vi "AMI Get 2D field (Polar).vi"(8 "error in":T2, 10 "Z-Axis Communications Config":T1={"GPIB address"=22, "GPIB bus"=0, "connection ID"=refnum, "IP"="192.168.2.200", "Active Comm Interface"=0, "Serial Port"="", "Programmer Type"=0} {"Programmer Type" items=["Model 430", "Model 420"]; "Active Comm Interface" items=["TCP/IP (Model 430 Only)", "RS232", "IEEE488"]}, 11 "Y-Axis Communications Config":T1={"GPIB address"=22, "GPIB bus"=0, "connection ID"=refnum, "IP"="192.168.2.200", "Active Comm Interface"=0, "Serial Port"="", "Programmer Type"=0} {"Programmer Type" items=["Model 430", "Model 420"]; "Active Comm Interface" items=["TCP/IP (Model 430 Only)", "RS232", "IEEE488"]}) -> (0 "error out":T2, 2 "phi (deg)":dbl min=0.0 format="%.3f", 3 "Radial (r) Field (T)":dbl min=0.0 format="%.3f")   [LabVIEW 2013]
panel:
  out "All Instruments Responded?":bool
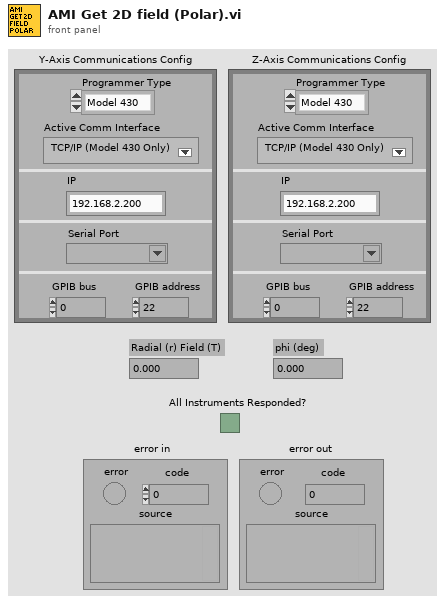
[diagram p1: front panel]
types:
  T1 = cluster{"GPIB address":i16, "GPIB bus":i16, "connection ID":refnum<k5>, "IP":string, "Active Comm Interface":u16, "Serial Port":refnum<visa-resource-name>, "Programmer Type":u16}
  T2 = cluster{"error":bool, "code":i32, "source":string}
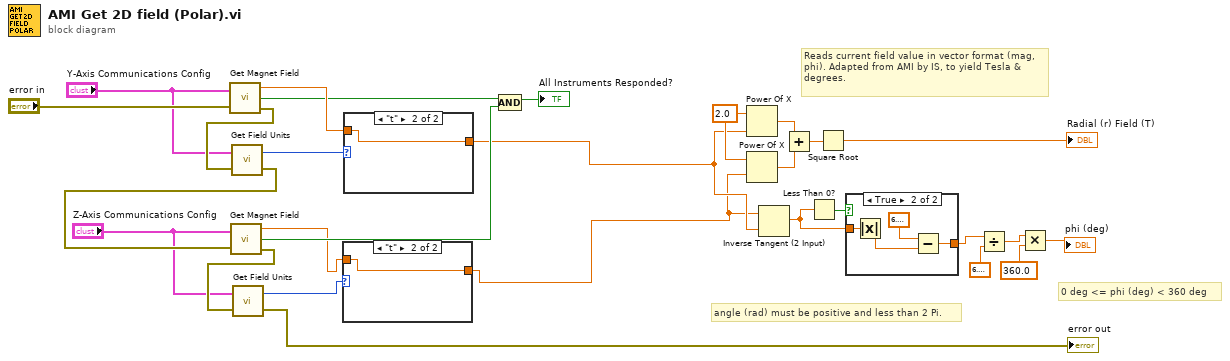
[diagram p0: block diagram]
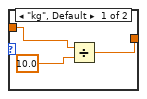
[diagram p2: hidden frame]
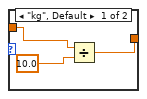
[diagram p4: hidden frame]
diagram:
  w16 = 2.0 ("y")
  # "Reads current field value in vector format (mag, phi). Adapted from AMI by IS, to yield Tesla & degrees."
  # "0 deg <= phi (deg) < 360 deg"
  # "angle (rad) must be positive and less than 2 Pi."
  n1 = call <userlib>:"Get Magnet Field.vi"("Communications Config"="Y-Axis Communications Config", "error in"="error in") -> ("Magnet Field (kG)"=w25:dbl, "Instrument Responded?"=w22:bool, "error out"=w27:T2)
  n2 = call <userlib>:"Get Field Units.vi"("error in"=w27, "Communications Config"="Y-Axis Communications Config") -> ("error out"=w23:T2, "Field Units"=w26:enum16{"kg", "t"})
  n3 = call <userlib>:"Get Magnet Field.vi"("Communications Config"="Z-Axis Communications Config", "error in"=w23) -> ("Magnet Field (kG)"=w8:dbl, "Instrument Responded?"=w21:bool, "error out"=w24:T2)
  n4 = call <userlib>:"Get Field Units.vi"("error in"=w24, "Communications Config"="Z-Axis Communications Config") -> ("error out"=→"error out":T2, "Field Units"=w7:enum16{"kg", "t"})
  n5 = case shown="\"t\"" w7 {
    tunnel: w8 -> [w29 w32]
    tunnel: [w30 w32] -> w6
    frame "kg", Default {
      n6 = Divide(x=w29, y=10.0) -> (x/y=w30:dbl)
    }
    frame "t" {
    }
  }
  n7 = case shown="\"t\"" w26 {
    tunnel: w25 -> [w33 w36]
    tunnel: [w34 w36] -> w9
    frame "kg", Default {
      n8 = Divide(x=w33, y=10.0) -> (x/y=w34:dbl)
    }
    frame "t" {
    }
  }
  n9 = Compound Arithmetic op=AND(w22, w21) -> (→"All Instruments Responded?":bool)
  n10 = Power Of X(1:w9, 2:w16) -> (0:w15:dbl)
  n11 = Power Of X(1:w6, 2:w16) -> (0:w14:dbl)
  n12 = Inverse Tangent (2 Input)(1:w9, 2:w6) -> (0:w11:dbl)
  n13 = Add(x=w15, y=w14) -> (x+y=w13:dbl)
  n14 = Less Than 0?(x=w11) -> (x < 0?=w12:bool)
  n15 = Square Root(x=w13) -> (sqrt(x)=→"Radial (r) Field (T)":dbl)
  n16 = case shown="True" w12 {
    tunnel: w11 -> [w37 w41]
    tunnel: [w37 w39] -> w5
    frame False {
    }
    frame True {
      n17 = Absolute Value(x=w41) -> (abs(x)=w40:dbl)
      n18 = Subtract(x=6.283185307179586, y=w40) -> (x-y=w39:dbl)
    }
  }
  n19 = Divide(x=w5, y=6.283185307179586) -> (x/y=w2:dbl)
  n20 = Multiply(x=w2, y=360.0) -> (x*y=→"phi (deg)":dbl)
